vi "Read Children.vi"(8 "Error In":errorcluster, 11 "NonTerminal In":refnum<class "NonTerminal.lvclass">) -> (0 "Error Out":errorcluster, 2 "Children":refnum<class "Abstract.lvclass">[](array[class]), 3 "NonTerminal Out":refnum<class "NonTerminal.lvclass">)   [LabVIEW 2018, in "Toolkit.lvlib" / "Nodes.lvlib" / "NonTerminal.lvclass"]
uses:
  NonTerminal.lvclass
  Abstract/Abstract.lvclass
  NonTerminal.lvclass/NonTerminal.ctl
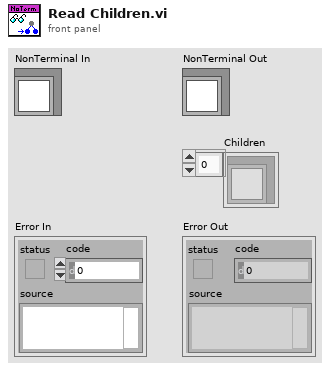
[diagram p1: front panel]
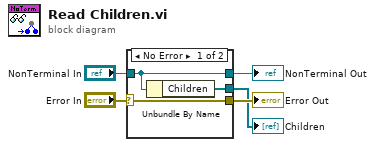
[diagram p0: block diagram]
diagram:
  n1 = case shown="No Error" "Error In" {
    selector: "Error In" -> [w8 w10]
    tunnel: [w8 w10] -> w4
    tunnel: [w7 w9] -> w2
    tunnel: "NonTerminal In" -> [w7 w9]
    tunnel: [w6 _] -> w1
    frame No Error {
      n2 = Unbundle By Name(w7) -> ("Children"=w6:refnum<class "Abstract.lvclass">[])
    }
    frame Error {
    }
  }
  "Error Out" <- w4
  "NonTerminal Out" <- w2
  "Children" <- w1
